vi "SECoP-addModule.vi"(6 "description":string, 7 "interface class(es)":string[](array[string]), 8 "error in (no error)":errorcluster, 10 "module name":string, 11 "DLL path (in)":T1) -> (0 "error out":errorcluster, 3 "DLL path (out)":T1)   [LabVIEW 2023, in "SECoP.lvlib"]
doc: "Call <b>\"SECoP-addModule.vi\"</b> to create a SECoP module inside the last created SECoP node.\n\n<b>DLL path</b> input and output of cluster from \"SECoP-Initialize.vi\"\n<b>module name</b> name of module\n<b>interface class(es)</b> supported interface class/-es (data type of command, see SECoP specification)\n<b>description</b> human readable description of this module"
uses:
  SECoP.lvlib
  SECoP-libraries.ctl
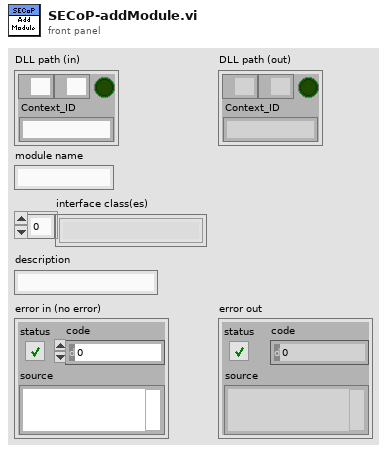
[diagram p1: front panel]
types:
  T1 = typedef "SECoP.lvlib/SECoP-libraries.ctl" = cluster{"serverDLL":path, "variantDLL":path, "cleanup_mode":bool, "Context_ID":string}
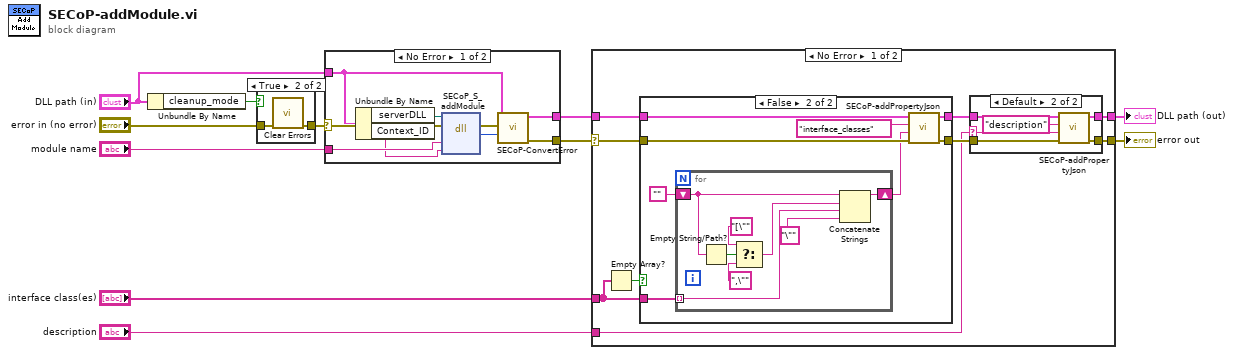
[diagram p0: block diagram]
diagram:
  n1 = Unbundle By Name("DLL path (in)") -> ("cleanup_mode"=w10:bool)
  n2 = case shown="True" w10 {
    tunnel: "error in (no error)" -> [w12 w14]
    tunnel: [w12 w13] -> w8
    frame False {
    }
    frame True {
      n3 = call <vilib>:"Clear Errors.vi"("error in (no error)"=w14) -> ("error out"=w13:errorcluster)  [unwired: 5 in, 1 out]
    }
  }
  n4 = case shown="No Error" w8 {
    selector: w8 -> [w21 w24]
    tunnel: "DLL path (in)" -> [w17 w25]
    tunnel: [w22 w25] -> w5
    tunnel: [w23 w24] -> w4
    tunnel: "module name" -> [w18 _]
    frame No Error {
      n5 = Unbundle By Name(w17) -> ("serverDLL"=w16:path, "Context_ID"=w15:string)
      n6 = dll-call lib="C:/Users/user/Desktop/x86_64/SECoP64.dll" fn="SECoP_S_addModule"(path in=w16, error in=w21, "name"=w18, "szContextID"=w15) -> (error out=w20:errorcluster, "return type"=w19:i32)  [unwired: 3 in, 1 out]
      n7 = call "SECoP-ConvertError.vi"("return code"=w19, "error in (no error)"=w20, "DLL path (in)"=w17) -> ("error out"=w23:errorcluster, "DLL path (out)"=w22:T1)  [unwired: 7 in]
    }
    frame Error {
    }
  }
  n8 = case shown="No Error" w4 {
    selector: w4 -> [w32 w62]
    tunnel: w5 -> [w33 w61]
    tunnel: [w28 w62] -> w2
    tunnel: [w29 w61] -> w3
    tunnel: "description" -> [w31 _]
    tunnel: "interface class(es)" -> [w27 _]
    frame No Error {
      n9 = Empty Array?(array=w27) -> (empty?=w26:bool)
      n10 = case shown="False" w26 {
        tunnel: w33 -> [w36 w44]
        tunnel: w32 -> [w35 w43]
        tunnel: [w35 w42] -> w34
        tunnel: [w36 w41] -> w30
        tunnel: w27 -> [_ w38]
        frame True {
        }
        frame False {
          n11 = for {
            tunnel: w38 -> [w46] mode=indexing
            shift-right: [w48] -> w37
            shift-left: "" -> [w47]
            n12 = Empty String/Path?(string/path=w47) -> (empty?=w52:bool)
            n13 = Select(t="[\"", s=w52, f=",\"") -> (s? t:f=w49:string)
            n14 = Concatenate Strings(w47, w49, w46, "\"") -> (w48:string)
          }
          n15 = call "SECoP-addPropertyJson.vi"("error in (no error)"=w43, "property value"=w37, "property name"="interface_classes", "DLL path (in)"=w44) -> ("error out"=w42:errorcluster, "DLL path (out)"=w41:T1)  [unwired: 6 in]
        }
      }
      n16 = case shown="Default" w31 {
        selector: w31 -> [_ w56]
        tunnel: w30 -> [w54 w60]
        tunnel: w34 -> [w53 w59]
        tunnel: [w53 w58] -> w28
        tunnel: [w54 w57] -> w29
        frame "" {
        }
        frame Default {
          n17 = call "SECoP-addPropertyJson.vi"("error in (no error)"=w59, "property value"=w56, "property name"="description", "DLL path (in)"=w60) -> ("error out"=w58:errorcluster, "DLL path (out)"=w57:T1)  [unwired: 6 in]
        }
      }
    }
    frame Error {
    }
  }
  "DLL path (out)" <- w3
  "error out" <- w2
